vi "Create 7z.bat Script.vi"(8 "error in (no error)":errorcluster, 11 "PostBuildSupport in":refnum<class "PostBuildSupport.lvclass">) -> (0 "error out":errorcluster, 2 "resulting string":string, 3 "PostBuildSupport out":refnum<class "PostBuildSupport.lvclass">)   [LabVIEW 2019, in "PostBuildSupport.lvclass"]
uses:
  PostBuildSupport.lvclass
  PostBuildSupport.lvclass/PostBuildSupport.ctl
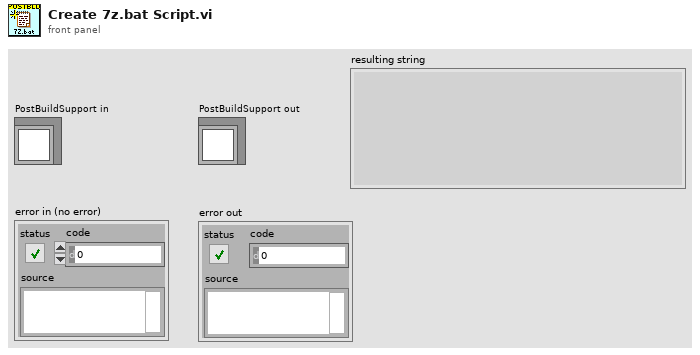
[diagram p1: front panel]
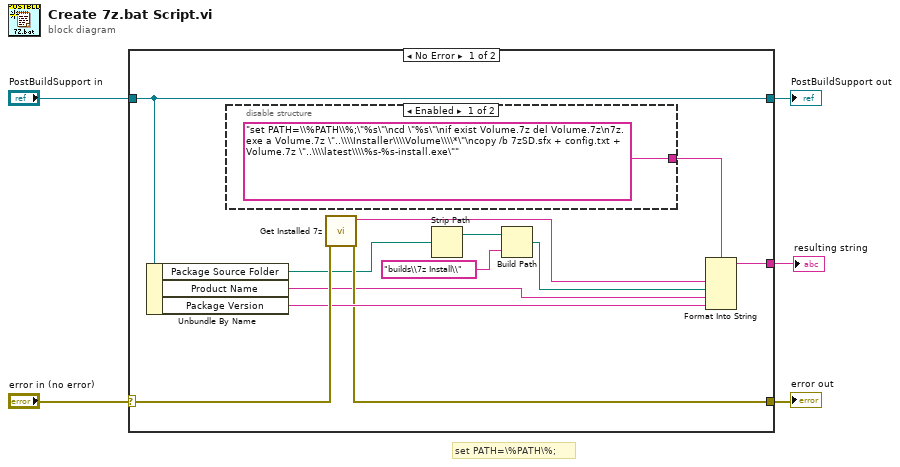
[diagram p0: block diagram]
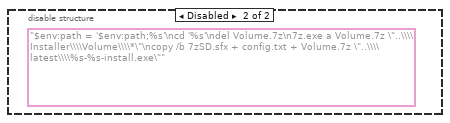
[diagram p2: hidden frame]
diagram:
  # "set PATH=\\%PATH\\%;"
  n1 = case shown="No Error" "error in (no error)" {
    selector: "error in (no error)" -> [w14 w20]
    tunnel: [w12 w20] -> w5
    tunnel: "PostBuildSupport in" -> [w15 w19]
    tunnel: [w15 w19] -> w2
    tunnel: [w11 _] -> w1
    frame No Error {
      n2 = Unbundle By Name(w15) -> ("Package Source Folder"=w8:path, "Product Name"=w6:string, "Package Version"=w13:string)
      n3 = disable-structure shown="Enabled" {
        disable-tunnel: ["set PATH=\\%PATH\\%;\"%s\"\ncd \"%s\"\nif exist Volume.7z del Volume.7z\n7z.exe a Volume.7z \"..\\\\Installer\\\\Volume\\\\*\"\ncopy /b 7zSD.sfx + config.txt + Volume.7z \"..\\\\latest\\\\%s-%s-install.exe\"" ("Name of target (My Computer)") _] -> w9
        frame Enabled {
        }
        frame Disabled {
          (unwired) "$env:path = '$env:path;%s'\ncd '%s'\ndel Volume.7z\n7z.exe a Volume.7z \"..\\\\Installer\\\\Volume\\\\*\"\ncopy /b 7zSD.sfx + config.txt + Volume.7z \"..\\\\latest\\\\%s-%s-install.exe\"" ("Name of target (My Computer)")
        }
      }
      n4 = call "Get Installed 7z.vi"("error in (no error)"=w14) -> ("error out"=w12:errorcluster, "Application Path"=w10:string)  [unwired: 9 in]
      n5 = Strip Path(path=w8) -> (stripped path=w17:path)  [unwired: 1 out]
      n6 = Build Path(base path=w17, name or relative path="builds\\7z Install\\") -> (appended path=w7:path)
      n7 = Format Into String(format string=w9, w10, w7, w6, w13) -> (resulting string=w11:string)  [unwired: 2 in, 1 out]
    }
    frame Error {
    }
  }
  "error out" <- w5
  "PostBuildSupport out" <- w2
  "resulting string" <- w1
